vi "Write Amount 1.vi"(8 "error in (no error)":errorcluster, 10 "Amount":dbl, 11 "AIncome in":refnum<class "AIncome.lvclass">) -> (0 "error out":errorcluster, 3 "AIncome out":refnum<class "AIncome.lvclass">)   [LabVIEW 2020, in "AIncome.lvclass"]
uses:
  AIncome.lvclass
  AIncome.lvclass/AIncome.ctl
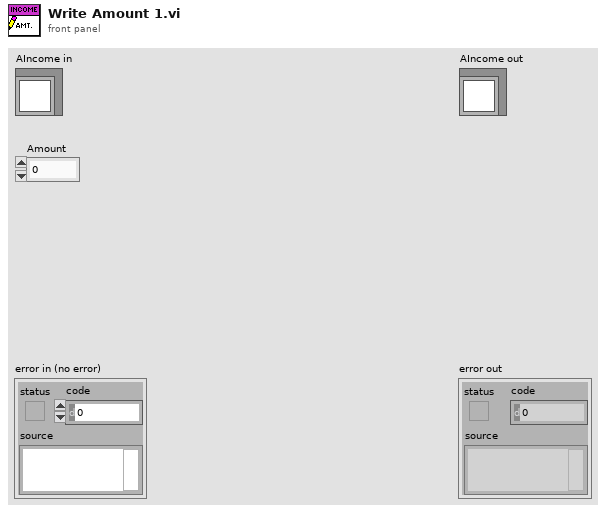
[diagram p1: front panel]
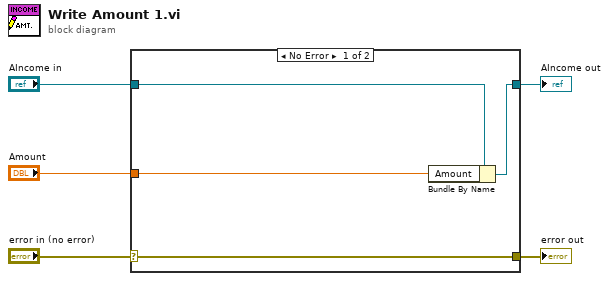
[diagram p0: block diagram]
diagram:
  n1 = case shown="No Error" "error in (no error)" {
    selector: "error in (no error)" -> [w9 w10]
    tunnel: [w9 w10] -> w4
    tunnel: [w7 w11] -> w2
    tunnel: "AIncome in" -> [w8 w11]
    tunnel: "Amount" -> [w6 _]
    frame No Error {
      n2 = Bundle By Name(cluster=w8, "Amount"=w6) -> (w7:refnum<class "AIncome.lvclass">)
    }
    frame Error {
    }
  }
  "error out" <- w4
  "AIncome out" <- w2
